vi "File Name Check.vi"(1 "File Name":string="你好啊") -> (0 "OK?":bool)   [LabVIEW 2020]
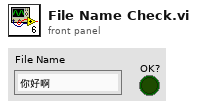
[diagram p1: front panel]
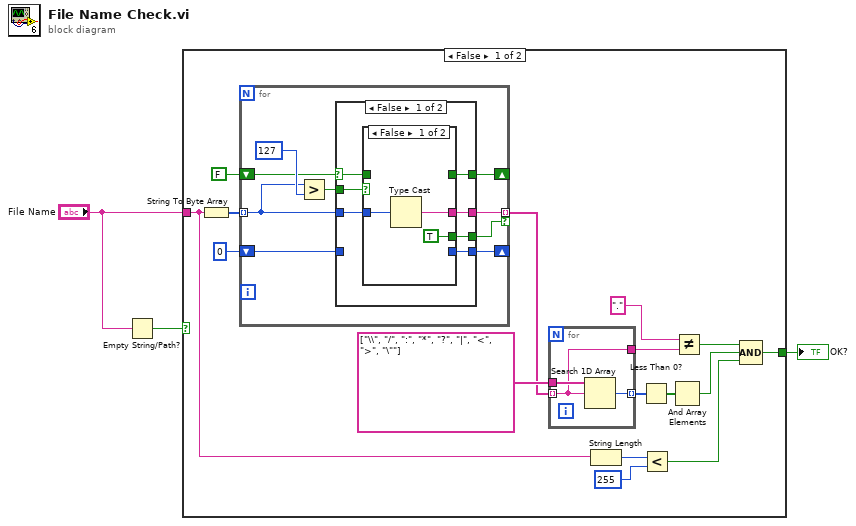
[diagram p0: block diagram]
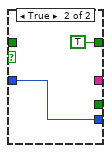
[diagram p2: hidden frame]
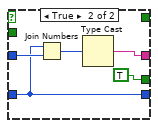
[diagram p3: hidden frame]
diagram:
  n1 = Empty String/Path?(string/path="File Name") -> (empty?=w1:bool)
  n2 = case shown="False" w1 {
    tunnel: [w9 _] -> w3
    tunnel: "File Name" -> [w7 _]
    frame False {
      n3 = String To Byte Array(string=w7) -> (unsigned byte array=w19:u8[])
      n4 = for {
        tunnel: w19 -> [w29] mode=indexing
        shift-right: [w25] -> _
        shift-left: FALSE -> [w28]
        shift-right: [w27] -> _
        shift-left: u8 0 -> [w26]
        tunnel: [w24] -> w8 mode=indexing if=w23
        n5 = Greater?(x=w29, y=u8 127) -> (0:w30:bool)
        n6 = case shown="False" w28 {
          selector: w28 -> [w35 _]
          tunnel: w30 -> [w38 _]
          tunnel: w29 -> [w37 w48]
          tunnel: [w36 w47] -> w27
          tunnel: w26 -> [_ w47]
          tunnel: [w34 _] -> w25
          tunnel: [w33 w45] -> w24
          tunnel: [w32 TRUE] -> w23
          frame False {
            n7 = case shown="False" w38 {
              tunnel: w37 -> [w41 w43]
              tunnel: [_ w43] -> w36
              tunnel: w35 -> [_ _]
              tunnel: [_ TRUE] -> w34
              tunnel: [w40 _] -> w33
              tunnel: [TRUE _] -> w32
              frame False {
                n8 = Type Cast(x=w41) -> (*(type *) &x=w40:string)  [unwired: 1 in]
              }
              frame True {
              }
            }
          }
          frame True {
            n9 = Join Numbers(hi=w47, lo=w48) -> ((hi.lo)=w46:u16)
            n10 = Type Cast(x=w46) -> (*(type *) &x=w45:string)  [unwired: 1 in]
          }
        }
      }
      n11 = for {
        tunnel: w8 -> [w20] mode=indexing
        tunnel: string[] ["\\", "/", ":", "*", "?", "|", "<", ">", "\""] -> [w22]
        tunnel: [w21] -> w15 mode=indexing
        tunnel: [w20] -> w13
        n12 = Search 1D Array(1D array=w22, element=w20) -> (index of element=w21:i32)  [unwired: 1 in]
      }
      n13 = String Length(string=w7) -> (length=w6:i32)
      n14 = Less Than 0?(x=w15) -> (x < 0?=w14:bool[])
      n15 = Less?(x=w6, y=255) -> (x < y?=w4:bool)
      n16 = And Array Elements(Boolean array=w14) -> (logical AND=w10:bool)
      n17 = Not Equal?(x=".", y=w13) -> (x != y?=w11:bool)
      n18 = Compound Arithmetic op=AND(w11, w10, w4) -> (w9:bool)
    }
    frame True {
    }
  }
  "OK?" <- w3
